vi "FTW-Test-JSON-IntegerOverflow.vi"() -> (0 "Test Result":errorcluster)   [LabVIEW 2015]
uses:
  src/json/core/FTW-JSON-Core-Type.ctl
  src/reflection/FTW-Reflection-Types.ctl
  src/json/FTW-JSON-Construct-FromBuffer.vi
  lib/FTW-KernelFilepath.vi
  codegen/xnode/json/fetch/FTW-JSON-Core-GetFlattenedValue.vi
  src/error/FTW-ERR-ThrowInvalidReferenceError.vi
  src/json/core/FTW-JSON-Core-ElementType.vi
  src/json/FTW-JSON-SerializeAndDestroy.vi
  src/json/core/FTW-JSON-Core-NumericType.vi
  src/error/FTW-ERR-ThrowError.vi
  codegen/xnode/FTW-JSON-Fetch.xnode
  src/json/FTW-JSON-Type.ctl
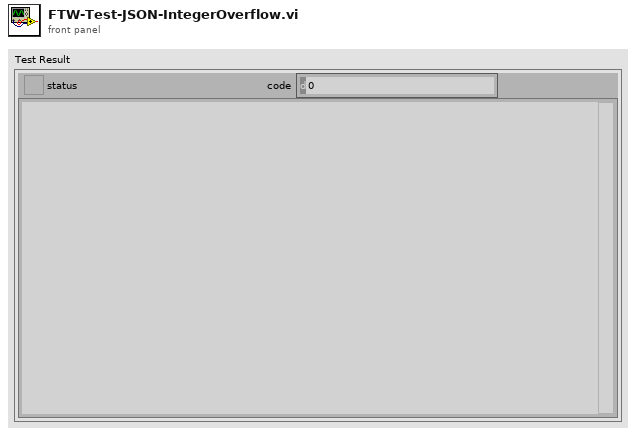
[diagram p1: front panel]
types:
  T1 = cluster{"Val":i8, "Val":i16, "Val":i32, "Val":i64, "Val":u8, "Val":u16, "Val":u32, "Val":u64}
  T2 = cluster{string, cluster{"I8":i8, "I16":i16, "I32":i32, "I64":i64, "U8":u8, "U16":u16, "U32":u32, "U64":u64}}[]
  T3 = typedef "FTW-JSON-Core-Type.ctl" = enum8{"Object", "Array", "String", "Integer", "Floating Point", "true", "false", "null", "undefined"}
  T4 = cluster{"I8":i8, "I16":i16, "I32":i32, "I64":i64, "U8":u8, "U16":u16, "U32":u32, "U64":u64}
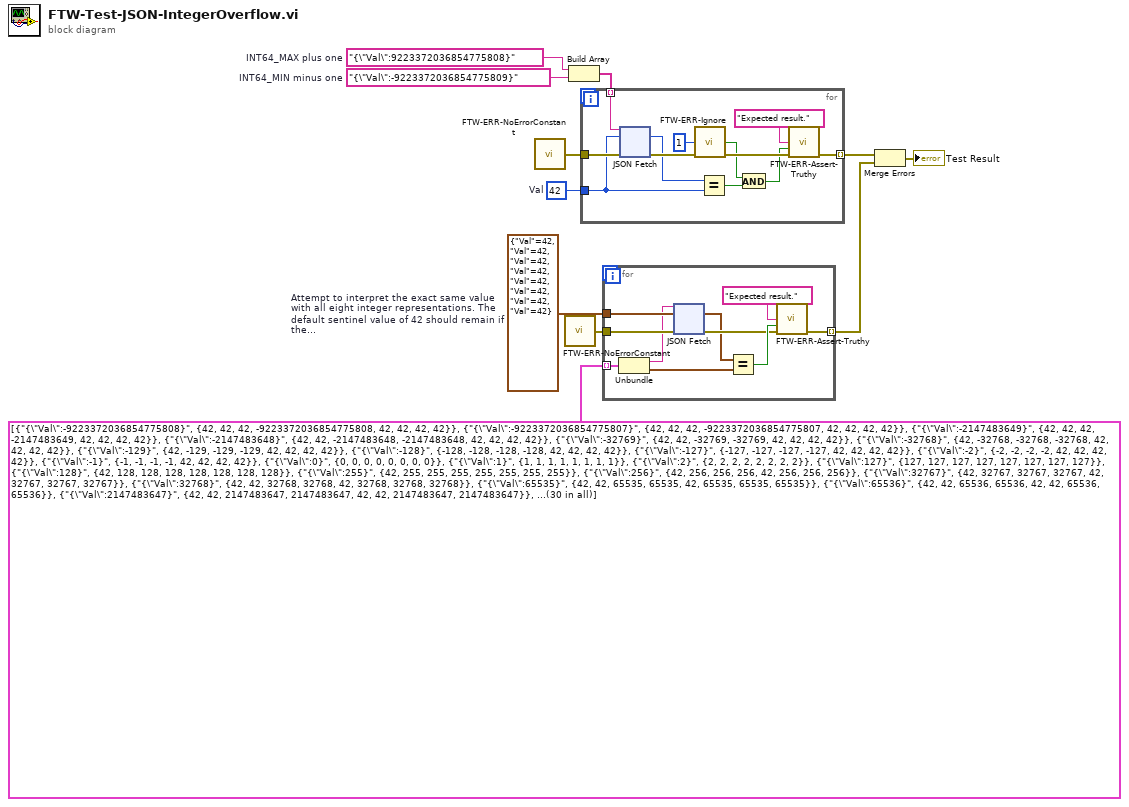
[diagram p0: block diagram]
diagram:
  w1 = i64 42  # Val
  w3 = "{\"Val\":-9223372036854775809}"  # INT64_MIN minus one
  w4 = "{\"Val\":9223372036854775808}"  # INT64_MAX plus one
  w7 = T1 {"Val"=42, "Val"=42, "Val"=42, "Val"=42, "Val"=42, "Val"=42, "Val"=42, "Val"=42}  # Attempt to interpret the exact same value with all eight integer representations. The default sentinel value of 42 should remain if the JSON value cannot be losslessly interpreted and represented by the capacity of the integer.
  n1 = call "FTW-ERR-NoErrorConstant.vi"() -> ("no error"=w6:errorcluster)
  n2 = call "FTW-ERR-NoErrorConstant.vi"() -> ("no error"=w11:errorcluster)
  n3 = Build Array(w4, w3) -> (w2:string[])
  n4 = for {
    tunnel: w6 -> [w23]
    tunnel: w2 -> [w22] mode=indexing
    tunnel: w1 -> [w12]
    tunnel: [w18] -> w5 mode=indexing
    n5 = xnode "JSON Fetch"("JSON"=w22, "Element Type and Default Value"=w12, "error in"=w23) -> ("Value"=w13:i64, "error out"=w19:errorcluster)  [unwired: 2 in, 3 out]
    n6 = call "FTW-ERR-Ignore.vi"("Error Code"=1, "error in"=w19) -> ("Error Cleared?"=w16:bool, "error out"=w17:errorcluster)  [unwired: 12 in]
    n7 = Equal?(x=w13, y=w12) -> (x = y?=w14:bool)
    n8 = And(x=w16, y=w14) -> (x .and. y?=w15:bool)
    n9 = call "FTW-ERR-Assert-Truthy.vi"("Assertion"="Expected result.", "Assertion holds true?"=w15, "error in"=w17) -> ("error out"=w18:errorcluster)  [unwired: 12 in]
  }
  n10 = for {
    tunnel: T2 [{"{\"Val\":-9223372036854775808}", {"I8"=42, "I16"=42, "I32"=42, "I64"=-9223372036854775808, "U8"=42, "U16"=42, "U32"=42, "U64"=42}}, {"{\"Val\":-9223372036854775807}", {"I8"=42, "I16"=42, "I32"=42, "I64"=-9223372036854775807, "U8"=42, "U16"=42, "U32"=42, "U64"=42}}, {"{\"Val\":-2147483649}", {"I8"=42, "I16"=42, "I32"=42, "I64"=-2147483649, "U8"=42, "U16"=42, "U32"=42, "U64"=42}}, {"{\"Val\":-2147483648}", {"I8"=42, "I16"=42, "I32"=-2147483648, "I64"=-2147483648, "U8"=42, "U16"=42, "U32"=42, "U64"=42}}, {"{\"Val\":-32769}", {"I8"=42, "I16"=42, "I32"=-32769, "I64"=-32769, "U8"=42, "U16"=42, "U32"=42, "U64"=42}}, {"{\"Val\":-32768}", {"I8"=42, "I16"=-32768, "I32"=-32768, "I64"=-32768, "U8"=42, "U16"=42, "U32"=42, "U64"=42}}, {"{\"Val\":-129}", {"I8"=42, "I16"=-129, "I32"=-129, "I64"=-129, "U8"=42, "U16"=42, "U32"=42, "U64"=42}}, {"{\"Val\":-128}", {"I8"=-128, "I16"=-128, "I32"=-128, "I64"=-128, "U8"=42, "U16"=42, "U32"=42, "U64"=42}}, {"{\"Val\":-127}", {"I8"=-127, "I16"=-127, "I32"=-127, "I64"=-127, "U8"=42, "U16"=42, "U32"=42, "U64"=42}}, {"{\"Val\":-2}", {"I8"=-2, "I16"=-2, "I32"=-2, "I64"=-2, "U8"=42, "U16"=42, "U32"=42, "U64"=42}}, {"{\"Val\":-1}", {"I8"=-1, "I16"=-1, "I32"=-1, "I64"=-1, "U8"=42, "U16"=42, "U32"=42, "U64"=42}}, {"{\"Val\":0}", {"I8"=0, "I16"=0, "I32"=0, "I64"=0, "U8"=0, "U16"=0, "U32"=0, "U64"=0}}, {"{\"Val\":1}", {"I8"=1, "I16"=1, "I32"=1, "I64"=1, "U8"=1, "U16"=1, "U32"=1, "U64"=1}}, {"{\"Val\":2}", {"I8"=2, "I16"=2, "I32"=2, "I64"=2, "U8"=2, "U16"=2, "U32"=2, "U64"=2}}, {"{\"Val\":127}", {"I8"=127, "I16"=127, "I32"=127, "I64"=127, "U8"=127, "U16"=127, "U32"=127, "U64"=127}}, {"{\"Val\":128}", {"I8"=42, "I16"=128, "I32"=128, "I64"=128, "U8"=128, "U16"=128, "U32"=128, "U64"=128}}, {"{\"Val\":255}", {"I8"=42, "I16"=255, "I32"=255, "I64"=255, "U8"=255, "U16"=255, "U32"=255, "U64"=255}}, {"{\"Val\":256}", {"I8"=42, "I16"=256, "I32"=256, "I64"=256, "U8"=42, "U16"=256, "U32"=256, "U64"=256}}, {"{\"Val\":32767}", {"I8"=42, "I16"=32767, "I32"=32767, "I64"=32767, "U8"=42, "U16"=32767, "U32"=32767, "U64"=32767}}, {"{\"Val\":32768}", {"I8"=42, "I16"=42, "I32"=32768, "I64"=32768, "U8"=42, "U16"=32768, "U32"=32768, "U64"=32768}}, {"{\"Val\":65535}", {"I8"=42, "I16"=42, "I32"=65535, "I64"=65535, "U8"=42, "U16"=65535, "U32"=65535, "U64"=65535}}, {"{\"Val\":65536}", {"I8"=42, "I16"=42, "I32"=65536, "I64"=65536, "U8"=42, "U16"=42, "U32"=65536, "U64"=65536}}, {"{\"Val\":2147483647}", {"I8"=42, "I16"=42, "I32"=2147483647, "I64"=2147483647, "U8"=42, "U16"=42, "U32"=2147483647, "U64"=2147483647}}, {"{\"Val\":2147483648}", {"I8"=42, "I16"=42, "I32"=42, "I64"=2147483648, "U8"=42, "U16"=42, "U32"=2147483648, "U64"=2147483648}}, {"{\"Val\":2147483649}", {"I8"=42, "I16"=42, "I32"=42, "I64"=2147483649, "U8"=42, "U16"=42, "U32"=2147483649, "U64"=2147483649}}, {"{\"Val\":4294967295}", {"I8"=42, "I16"=42, "I32"=42, "I64"=4294967295, "U8"=42, "U16"=42, "U32"=4294967295, "U64"=4294967295}}, {"{\"Val\":4294967296}", {"I8"=42, "I16"=42, "I32"=42, "I64"=4294967296, "U8"=42, "U16"=42, "U32"=42, "U64"=4294967296}}, {"{\"Val\":4294967297}", {"I8"=42, "I16"=42, "I32"=42, "I64"=4294967297, "U8"=42, "U16"=42, "U32"=42, "U64"=4294967297}}, {"{\"Val\":9223372036854775806}", {"I8"=42, "I16"=42, "I32"=42, "I64"=9223372036854775806, "U8"=42, "U16"=42, "U32"=42, "U64"=9223372036854775806}}, {"{\"Val\":9223372036854775807}", {"I8"=42, "I16"=42, "I32"=42, "I64"=9223372036854775807, "U8"=42, "U16"=42, "U32"=42, "U64"=9223372036854775807}}] -> [w89] mode=indexing
    tunnel: w11 -> [w84]
    tunnel: [w88] -> w9 mode=indexing
    tunnel: w7 -> [w83]
    n11 = Unbundle(w89) -> (w82:string, w80:T4)
    n12 = xnode "JSON Fetch"("JSON"=w82, "Element Type and Default Value"=w83, "error in"=w84) -> ("Value"=w81:T1, "error out"=w85:errorcluster)  [unwired: 2 in, 3 out]
    n13 = Equal?(x=w81, y=w80) -> (x = y?=w87:bool)
    n14 = call "FTW-ERR-Assert-Truthy.vi"("Assertion"="Expected result.", "Assertion holds true?"=w87, "error in"=w85) -> ("error out"=w88:errorcluster)  [unwired: 12 in]
  }
  n15 = Merge Errors(w5, w9) -> (→"Test Result":errorcluster)
